vi "FITS_LoadImgSGL.vi"(8 "error in":errorcluster, 11 "Interaction/Command Matrix File":path) -> (0 "error out":errorcluster, 2 "Image 2D":sgl[][](array[numeric]) format="%.2f", 3 "Image 1D":sgl[](array[numeric]))   [LabVIEW 2016]
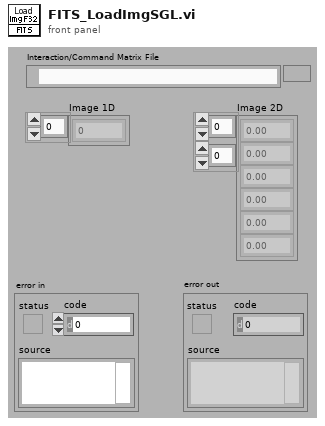
[diagram p1: front panel]
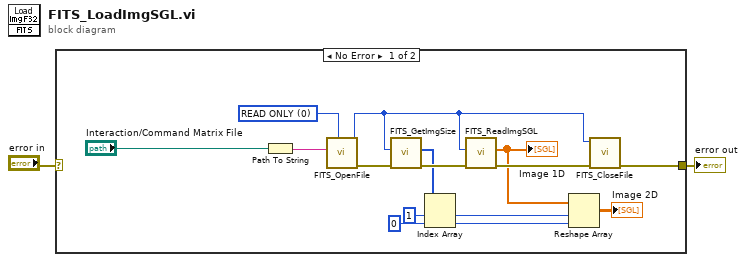
[diagram p0: block diagram]
diagram:
  n1 = case shown="No Error" "error in" {
    selector: "error in" -> [_ w18]
    tunnel: [w5 w18] -> w2
    frame No Error {
      w16 = 0 items=["READ ONLY", "READ/WRITE"] ("mode")
      n2 = Path To String(path="Interaction/Command Matrix File") -> (string=w17:string)
      n3 = call "FITS_OpenFile.vi"("mode"=w16, "filename"=w17) -> ("error out"=w14:errorcluster, "fp out"=w3:u64)  [unwired: 1 in, 7 out]
      n4 = call "FITS_GetImgSize.vi"("error in"=w14, "ref"=w3) -> ("error out"=w13:errorcluster, "Size"=w9:i32[])  [unwired: 8 out]
      n5 = Index Array(array=w9, index #1=1 ("index"), index #2=0 ("index")) -> (element #1=w8:i32, element #2=w7:i32)
      n6 = call "FITS_ReadImgSGL.vi"("error in"=w13, "ref"=w3) -> ("error out"=w15:errorcluster, "Img Data"=w4:sgl[])  [unwired: 8 in]
      "Image 1D" <- w4
      n7 = Reshape Array(w4, w8, w7) -> (→"Image 2D":sgl[][])
      n8 = call "FITS_CloseFile.vi"("error in"=w15, "ref in"=w3) -> ("error out"=w5:errorcluster)  [unwired: 1 in, 8 out]
    }
    frame Error {
    }
  }
  "error out" <- w2
